vi "dvp Vi Open By Name.vi"(9 "pHandle":u32, 10 "type":u32(ring) items=["OPEN_OFFLINE", "OPEN_NORMAL"], 11 "friendlyName":string) -> (1 "pHandle out":u32, 2 "function return":u32(ring), 3 "friendlyName out":string)   [LabVIEW 2018, in "LabViewDVPCamera.lvlib"]
doc: "LabviewDvp2Api dvpStatus dvpViOpenByName(char *friendlyName, dvpOpenMode type, dvpHandle *pHandle);"
uses:
  LabViewDVPCamera.lvlib
  LabViewDVPCamera/LabViewDVPCamera.dll
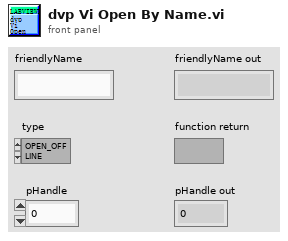
[diagram p1: front panel]
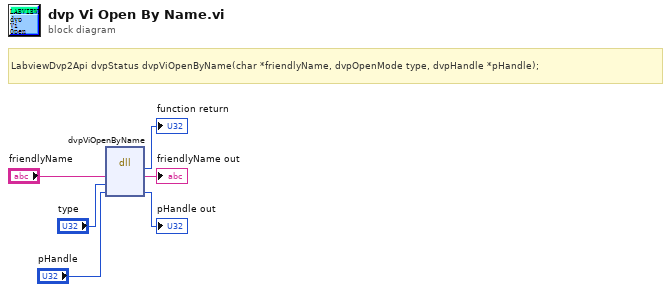
[diagram p0: block diagram]
diagram:
  # "LabviewDvp2Api dvpStatus dvpViOpenByName(char *friendlyName, dvpOpenMode type, dvpHandle *pHandle);"
  n1 = dll-call lib="C:/Program Files (x86)/DVP2 Labview cn 64/Sample/LabViewDVPCamera/LabViewDVPCamera.*" fn="dvpViOpenByName"("friendlyName"="friendlyName", "type"="type", "pHandle"="pHandle") -> (→"function return":u32, "friendlyName"=→"friendlyName out":string, "pHandle"=→"pHandle out":u32)  [unwired: 4 in, 2 out]
